vi "SaveVI.vi"(9 "queueOUT":refnum<queue>, 10 "queueIN":refnum<queue>) -> ()   [LabVIEW 2015, in "Control-Client.lvclass"]
uses:
  Control-Client.lvclass
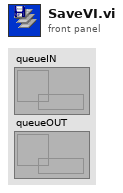
[diagram p1: front panel]
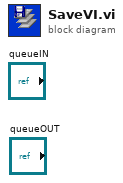
[diagram p0: block diagram]
diagram:
